vi "Serialize I2C Timestamp.vi"(0 "i2c monitor":T1 {"monitor word" format="%.0x"}, 5 "timestamp counter value":T2) -> (4 "data":fxp<+,58,58>, 6 "create timestamp":bool)   [LabVIEW 2020, in "GettingStarted_Common_148X_FPGA.lvlib"]
uses:
  GettingStarted_Common_148X_FPGA.lvlib
  <instrlib>/FlexRIO/CSI-2/v2/FPGA/Types/Timestamp Counter Value.ctl
  <instrlib>/FlexRIO/API/FPGA/v1/IO/NI148x/i2c monitor.ctl
  <instrlib>/FlexRIO/CSI-2/v2/FPGA/NI CSI-2 API FPGA v2.lvlib
  <instrlib>/FlexRIO/API/FPGA/v1/IO/NI148x/FlexRIO 148x FPGA v1.lvlib
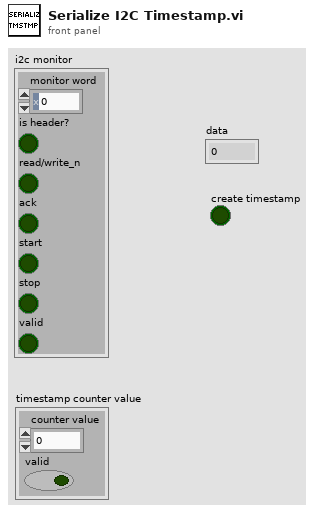
[diagram p1: front panel]
types:
  T1 = typedef "FlexRIO 148x FPGA v1.lvlib/i2c monitor.ctl" = cluster{"monitor word":u8, "is header?":bool, "read/write_n":bool, "ack":bool, "start":bool, "stop":bool, "valid":bool}
  T2 = typedef "NI CSI-2 API FPGA v2.lvlib/Timestamp Counter Value.ctl" = cluster{"counter value":u64, "valid":bool}
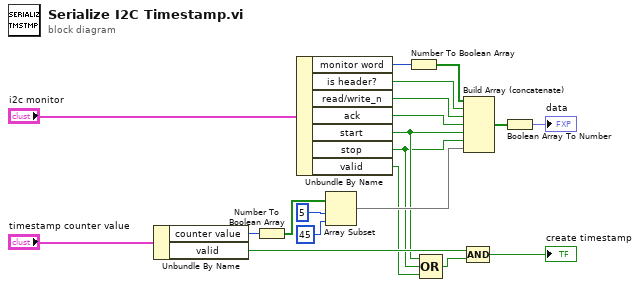
[diagram p0: block diagram]
diagram:
  n1 = Unbundle By Name("timestamp counter value") -> ("counter value"=w12:u64, "valid"=w19:bool)
  n2 = Number To Boolean Array(number=w12) -> (Boolean array=w11:bool[])
  n3 = Unbundle By Name("i2c monitor") -> ("monitor word"=w17:u8, "is header?"=w15:bool, "read/write_n"=w14:bool, "ack"=w13:bool, "start"=w5:bool, "stop"=w4:bool, "valid"=w3:bool)
  n4 = Array Subset(array=w11, index=5, length=45) -> (w8:bool[])
  n5 = Number To Boolean Array(number=w17) -> (Boolean array=w16:bool[])
  n6 = Compound Arithmetic op=OR(w5, w4, w3) -> (w2:bool)
  n7 = Build Array (concatenate)(w16, w15, w14, w13, w5, w4, w8) -> (w7:bool[])
  n8 = Compound Arithmetic op=AND(w19, w2) -> (→"create timestamp":bool)
  n9 = Boolean Array To Number(Boolean array=w7) -> (number=→"data":fxp<+,58,58>)
